vi "Get Parameter.vi"(8 "error in (no error)":errorcluster, 10 "Parameter name":string, 11 "TDCManager":T1) -> (0 "error out":errorcluster, 2 "Value":string, 3 "TDCManager":T1)   [LabVIEW 2016, in "HPTDC Driver Library.lvlib"]
uses:
  HPTDC Driver Library.lvlib
  Typedefs/TDCManager.ctl
  C:/Users/CRT Controller/CRTC Labview Application/Source/HPTDC Driver Library Folder/Library files/hptdc_net4_3.7.0_x64.dll
  hptdc_net4_3.7.0_x64.dll
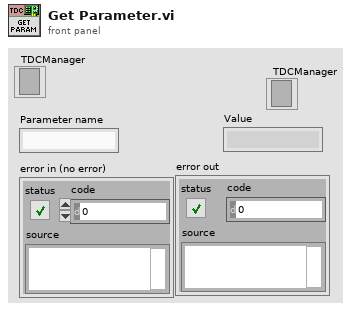
[diagram p1: front panel]
types:
  T1 = typedef "HPTDC Driver Library.lvlib/TDCManager.ctl" = refnum<k24>
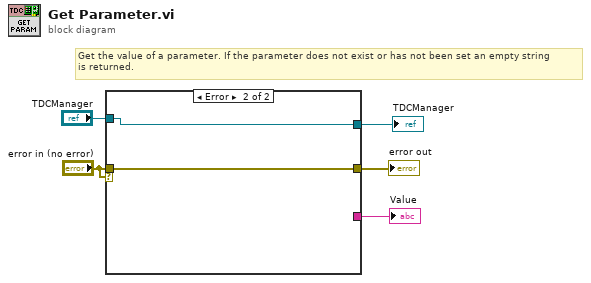
[diagram p0: block diagram]
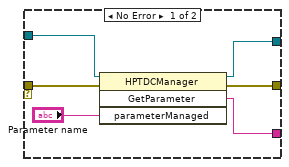
[diagram p2: hidden frame]
diagram:
  # "Get the value of a parameter. If the parameter does not exist or has not been set an empty string\nis returned."
  n1 = case shown="Error" "error in (no error)" {
    tunnel: "error in (no error)" -> [w11 w13]
    tunnel: [w10 w13] -> w5
    tunnel: [w9 w12] -> w4
    tunnel: "TDCManager" -> [w7 w12]
    tunnel: [w6 _] -> w2
    frame No Error {
      n2 = invoke class="HPTDCManager" method="GetParameter"(reference=w7, error in=w11, "parameterManaged"="Parameter name") -> (reference out=w9:T1, error out=w10:errorcluster, "GetParameter"=w6:string)  [unwired: 1 in, 1 out]
    }
    frame Error {
    }
  }
  "error out" <- w5
  "TDCManager" <- w4
  "Value" <- w2
